vi "SCMP Rotation and Focus Check.vi"(8 "error in":errorcluster, 11 "FITS Header In":T1={"Wavelength (nm)"=530.15, "Exposure (s)"=0.05, "Tuning Delay (ms)"=1000.0, "Beam Type (-1/1)"=1.0, "Tuning Voltages"=[1.111, 2.222, 3.333, 4.444], "Observer"="observer", "Light Shapping Diffuser"=enum."In Beam", "Comment"="", "Data Type"=enum."HOLE", "Mod Cycles"=0, "SCD Calibration Optics"=enum."1 - Polarizer @0, I+Q", "SCD Emission Line Filter"=enum."1-557.6nm", "Cookbook"="", "COMP-S Calibration Wheel"=enum."Dark", "COMP-S Andover Filter Wheel"=enum."530.3nm/HWB 0.34nm (Fe XIV)", "FOV Rotation (deg)"=66.0, "Objective Lens Position (mm)"=0.0, "Occulter size"=0.0, "Time End"=timestamp(3382374145.421875 s since 1904-01-01), "Acc Exposure (s)"=0.0, "Time Stamp Array"=[], "Camera Serial Number"=[], "Camera Temp"=[], "Camera PI (mm)"=[], "Time Start"=timestamp(3382374145.421875 s since 1904-01-01), "Peripherals"={"ILX controler"=FALSE, "Zone temperatures"=FALSE, "Andor"=FALSE, "Andor 2"=FALSE, "PI Stages"=FALSE, "AISAS mechanisms"=FALSE, "AISAS Mech.lvclass"=refnum, "Zone temp ref"=variant, "FWs"=FALSE}, "FITS paths"=[], "Cameras"=enum."Andor", "load preset cbk"=FALSE, "periodic check count"=0, "COMP-S Calibration Wheel 2"=enum."Dark", "Calib"=enum."Dark", "Abso Aperture"=66.0, "Nominal Aperture"=66.0, "Pointer IP"="127.0.0.1"} {"Nominal Aperture" format="%.1f"; "Abso Aperture" format="%.1f"; "Camera PI (mm)" format="%_3g"; "Acc Exposure (s)" format="%^.3g"; "Occulter size" format="%.2f"; "Objective Lens Position (mm)" min=70.0 max=152.0 format="%.2f"; "FOV Rotation (deg)" format="%.1f"; "Exposure (s)" format="%^.3g"; "Wavelength (nm)" format="%_6g"}) -> (0 "error out":errorcluster, 1 "Comment out":string="Test", 2 "Observer out":string="Observer", 3 "FITS Header Out":T1={"Wavelength (nm)"=530.15, "Exposure (s)"=0.05, "Tuning Delay (ms)"=1000.0, "Beam Type (-1/1)"=1.0, "Tuning Voltages"=[1.111, 2.222, 3.333, 4.444], "Observer"="observer", "Light Shapping Diffuser"=enum."In Beam", "Comment"="", "Data Type"=enum."HOLE", "Mod Cycles"=0, "SCD Calibration Optics"=enum."1 - Polarizer @0, I+Q", "SCD Emission Line Filter"=enum."1-557.6nm", "Cookbook"="", "COMP-S Calibration Wheel"=enum."Dark", "COMP-S Andover Filter Wheel"=enum."530.3nm/HWB 0.34nm (Fe XIV)", "FOV Rotation (deg)"=66.0, "Objective Lens Position (mm)"=0.0, "Occulter size"=0.0, "Time End"=timestamp(3382374145.421875 s since 1904-01-01), "Acc Exposure (s)"=0.0, "Time Stamp Array"=[], "Camera Serial Number"=[], "Camera Temp"=[], "Camera PI (mm)"=[], "Time Start"=timestamp(3382374145.421875 s since 1904-01-01), "Peripherals"={"ILX controler"=FALSE, "Zone temperatures"=FALSE, "Andor"=FALSE, "Andor 2"=FALSE, "PI Stages"=FALSE, "AISAS mechanisms"=FALSE, "AISAS Mech.lvclass"=refnum, "Zone temp ref"=variant, "FWs"=FALSE}, "FITS paths"=[], "Cameras"=enum."Andor", "load preset cbk"=FALSE, "periodic check count"=0, "COMP-S Calibration Wheel 2"=enum."Dark", "Calib"=enum."Dark", "Abso Aperture"=66.0, "Nominal Aperture"=66.0, "Pointer IP"="127.0.0.1"} {"Nominal Aperture" format="%.1f"; "Abso Aperture" format="%.1f"; "Camera PI (mm)" format="%_3g"; "Acc Exposure (s)" format="%^.3g"; "Occulter size" format="%.2f"; "Objective Lens Position (mm)" min=70.0 max=152.0 format="%.2f"; "FOV Rotation (deg)" format="%.1f"; "Exposure (s)" format="%^.3g"; "Wavelength (nm)" format="%_6g"}, 5 "Pointer IP":string)   [LabVIEW 2014]
uses:
  Controls/Diffuser.ctl
  Controls/SCMP observers.ctl
  Controls/SCD - FITS Cluster.ctl
  Mech/AISAS Mech.lvclass
  Controls/FITS Data type.ctl
  Controls/SCD - Calibration Optics Filter Wheel.ctl
  Controls/SCD - EDT - Emission Line Filter Wheel.ctl
  Controls/CoMP-S Controls/Polarization Optics Filter Wheel.ctl
  Controls/CoMP-S Controls/Emission Line Filter Wheel.ctl
  Controls/focus.ctl
  Controls/peripherals.ctl
  Controls/Cameras select.ctl
  <vilib>/Utility/xml.llb/Read From XML File(array).vi
panel:
  in  "Nominal Aperture":dbl=196.0 caption="Nominal aperture diameter [mm]" min=0.0 max=360.0 format="%.1f"
  in  "Abs Aperture":dbl=39.7 caption="Absolute calibration aperture diameter [mm]" min=0.0 max=360.0 format="%.1f"
  in  "Focus":dbl=103.0 min=70.0 max=152.0 format="%.2f"
  in  "Occulter size":dbl=103.0 format="%.2f"
  out "Generated XML":string
  in  "Observer":string="Observer"
  in  "Comment":string="Test"
  in  "Observer Enum":T11 items=["INY", "RYBAK", "SCHWARTZ", "HUTAR", "TREMBAC"]
  in  "Diffuser":T2=enum."In Beam"
  out "OBS_PROG OUT":string
  in  "Observer Program":u16(ring) items=["TEST", "OBS_PROG 001: SPEKTROPOLARIMETRIA POKOJNEJ PROTUBERANCIE A JEJ KAVITY - 854,656,637,530 (P.Schwartz)", "OBS_PROG 002: SPEKTROPOLARIMETRIA POKOJNEJ PROTUBERANCIE - 656 (Y.Su)", "OBS_PROG 003: SPEKTROPOLARIMETRIA PROTUBERANCII A KORONY - 656,587,530 (P.Schwartz)", "OBS_PROG 004: SPEKTROPOLARIMETRIA FILAMENTOV NA DISKU - 854,656,587 (P.Schwartz)", "OBS_PROG 005: SPEKTROPOLARIMETRIA PROTUBERANCII -s 854,656,587,530 (P.Schwartz)", "OBS_PROG 006: SPEKTROPOLARIMETRIA PROTUBERANCII A KORONY - 854,656,587,530 (P.Schwartz)", "CAL_PROG 001: CORONAGRAPH FOCUS DETERMINATION FOR ALL LINES", "TEST_PROG 001: DATA ACQUISITION BY CAMERAS"]
  out "Observer txt":string
  in  "Rotation Angle":dbl min=0.0 max=360.0 format="%.1f"
  in  "stop":bool
  # "Please check initial values !!!"
  # "motorized 39.7 mm, manual 40.0 mm"
  # "If values are right, then press OK"
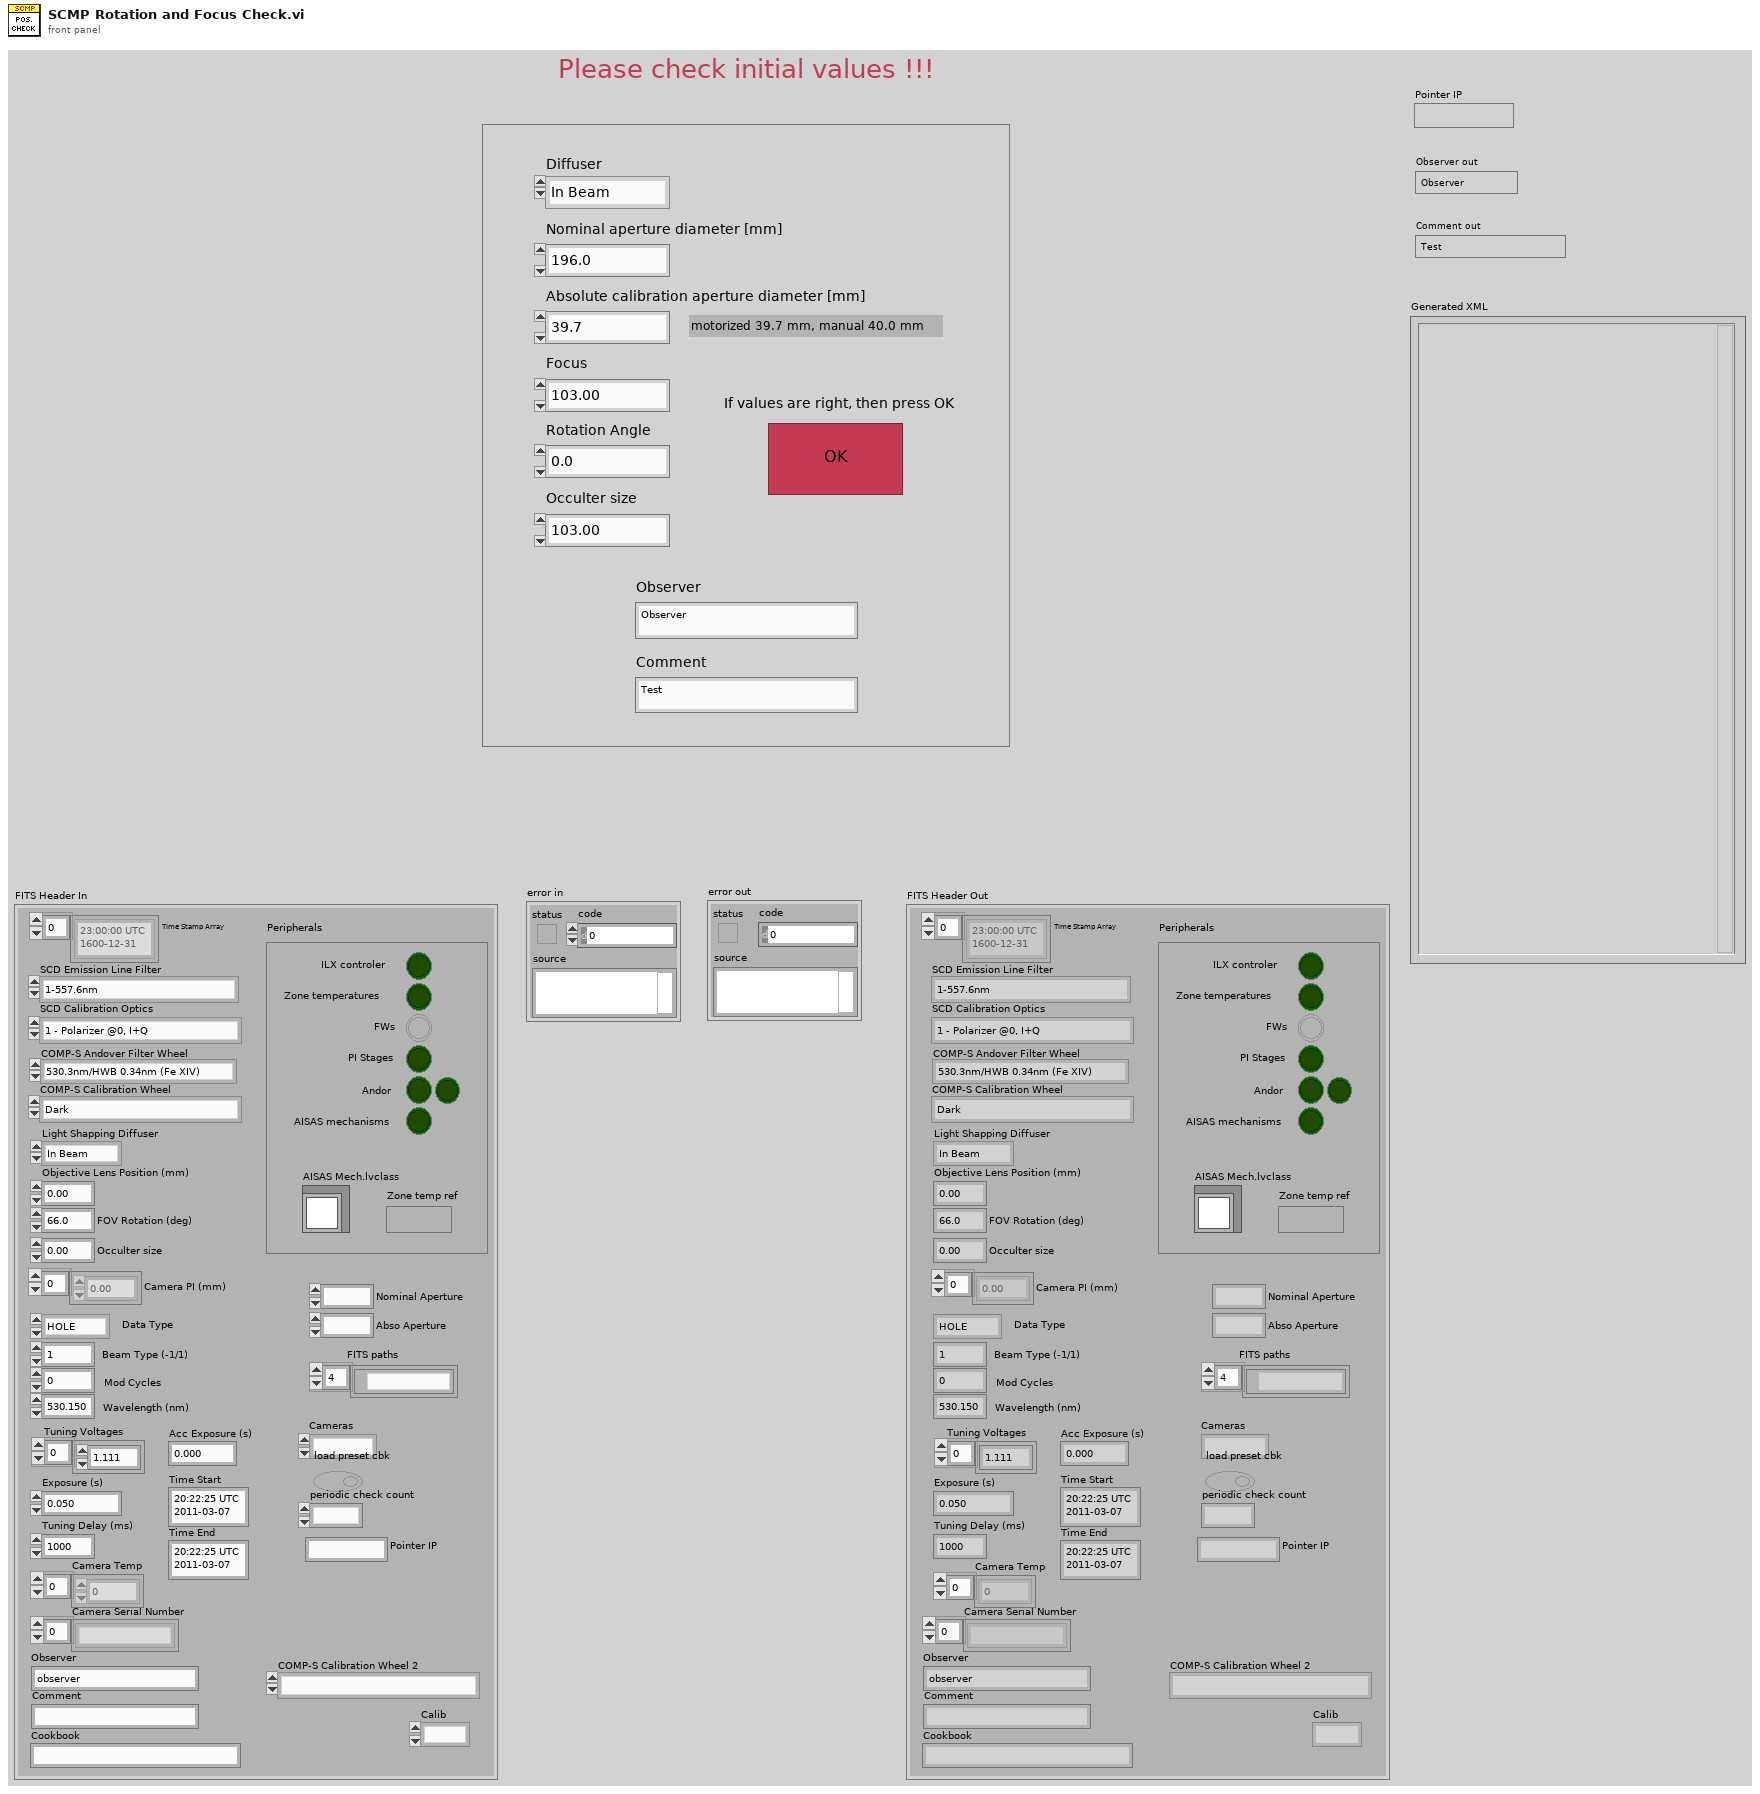
[diagram p1: front panel]
types:
  T1 = typedef "SCD - FITS Cluster.ctl" = cluster{"Wavelength (nm)":dbl, "Exposure (s)":dbl, "Tuning Delay (ms)":dbl, "Beam Type (-1/1)":dbl, "Tuning Voltages":dbl[], "Observer":string, "Light Shapping Diffuser":T2, "Comment":string, "Data Type":T3, "Mod Cycles":u16, "SCD Calibration Optics":T4, "SCD Emission Line Filter":T5, "Cookbook":string, "COMP-S Calibration Wheel":T6, "COMP-S Andover Filter Wheel":T7, "FOV Rotation (deg)":dbl, "Objective Lens Position (mm)":T8, "Occulter size":dbl, "Time End":timestamp, "Acc Exposure (s)":dbl, "Time Stamp Array":timestamp[], "Camera Serial Number":string[], "Camera Temp":dbl[], "Camera PI (mm)":dbl[], "Time Start":timestamp, "Peripherals":T9, "FITS paths":path[], "Cameras":T10, "load preset cbk":bool, "periodic check count":i32, "COMP-S Calibration Wheel 2":T6, "Calib":enum16{"Dark", "Flat"}, "Abso Aperture":dbl, "Nominal Aperture":dbl, "Pointer IP":string}
  T2 = typedef "Diffuser.ctl" = enum16{"Out of Beam", "In Beam"}
  T3 = typedef "FITS Data type.ctl" = enum16{"LIVE", "DARK", "FLAT", "CALI", "OBSE", "ABSO", "AURE", "TARG", "OBJE", "HOLE", "OREX", "THRO", "CHIP"}
  T4 = typedef "SCD - Calibration Optics Filter Wheel.ctl" = enum16{"1 - Polarizer @0, I+Q", "2 - Polarizer @90, I-Q", "3 - Polarizer @45, I+U", "4 - Polarizer @135, I-U", "5 - Polarizer @0, Retarder @45, I+V", "6 - Polarizer @0, Retarder @135, I-V", "7 - Dark", "8 - Clear", "9 - N/A"}
  T5 = typedef "SCD - EDT - Emission Line Filter Wheel.ctl" = enum16{"1-557.6nm", "2-587.6nm", "3-589.6nm", "4-630.2nm", "5-656.4nm", "6-849.8nm", "7-854.2nm", "8-866.2nm", "9-1083.0nm"}
  T6 = typedef "Polarization Optics Filter Wheel.ctl" = enum16{"Dark", "Clear", "Exchange Lens", "Polarizer @0, I+Q", "Polarizer @90, I-Q", "Polarizer @45, I+U", "Polarizer @135, I-U", "Polarizer @0, Retarder @45, I+V", "Polarizer @0, Retarder @135, I-V"}
  T7 = typedef "Emission Line Filter Wheel.ctl" = enum16{"530.3nm/HWB 0.34nm (Fe XIV)", "587.6nm/HBW 0.44nm (He I D3)", "637.5nm/HBW 0.53nm (Fe X)", "656.3nm/HBW 0.57nm (H-Alpha)", "789.2nm/HBW 0.85nm (Fe XI)", "854.2nm/HBW 1.01nm (Ca I)", "1074.7nm/HBW 2.34nm (Fe XIII)", "1079.8nm/HBW 1.64nm (Fe XIII)", "1083.0nm/HBW 1.66nm (He I)"}
  T8 = typedef "focus.ctl" = dbl
  T9 = typedef "peripherals.ctl" = cluster{"ILX controler":bool, "Zone temperatures":bool, "Andor":bool, "Andor 2":bool, "PI Stages":bool, "AISAS mechanisms":bool, "AISAS Mech.lvclass":refnum<class "AISAS Mech.lvclass">, "Zone temp ref":variant, "FWs":bool}
  T10 = typedef "Cameras select.ctl" = enum16{"Andor", "GDR"}
  T11 = typedef "SCMP observers.ctl" = u16
  T12 = enum8{"Enabled", "Disabled", "Disabled and Grayed Out"}
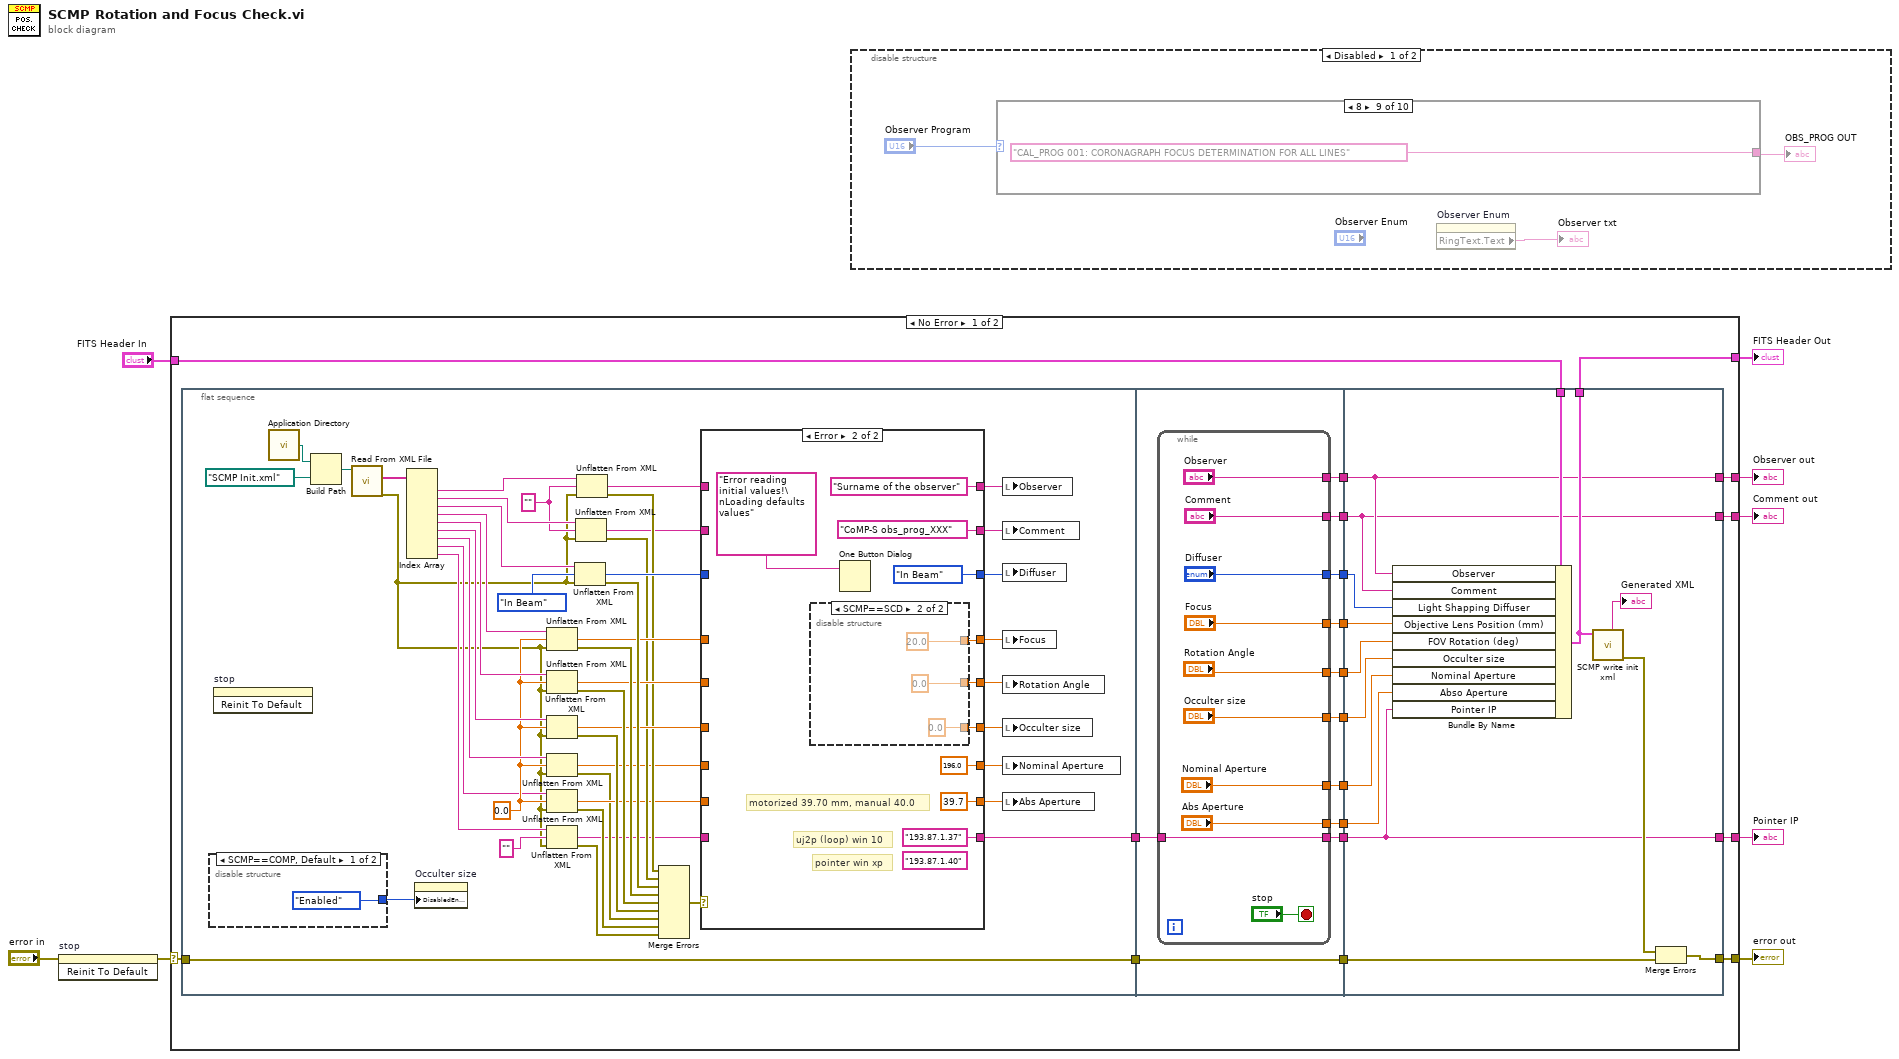
[diagram p0: block diagram]
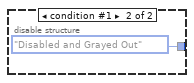
[diagram p2: hidden frame]
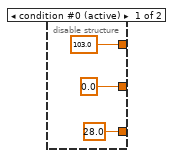
[diagram p4: hidden frame]
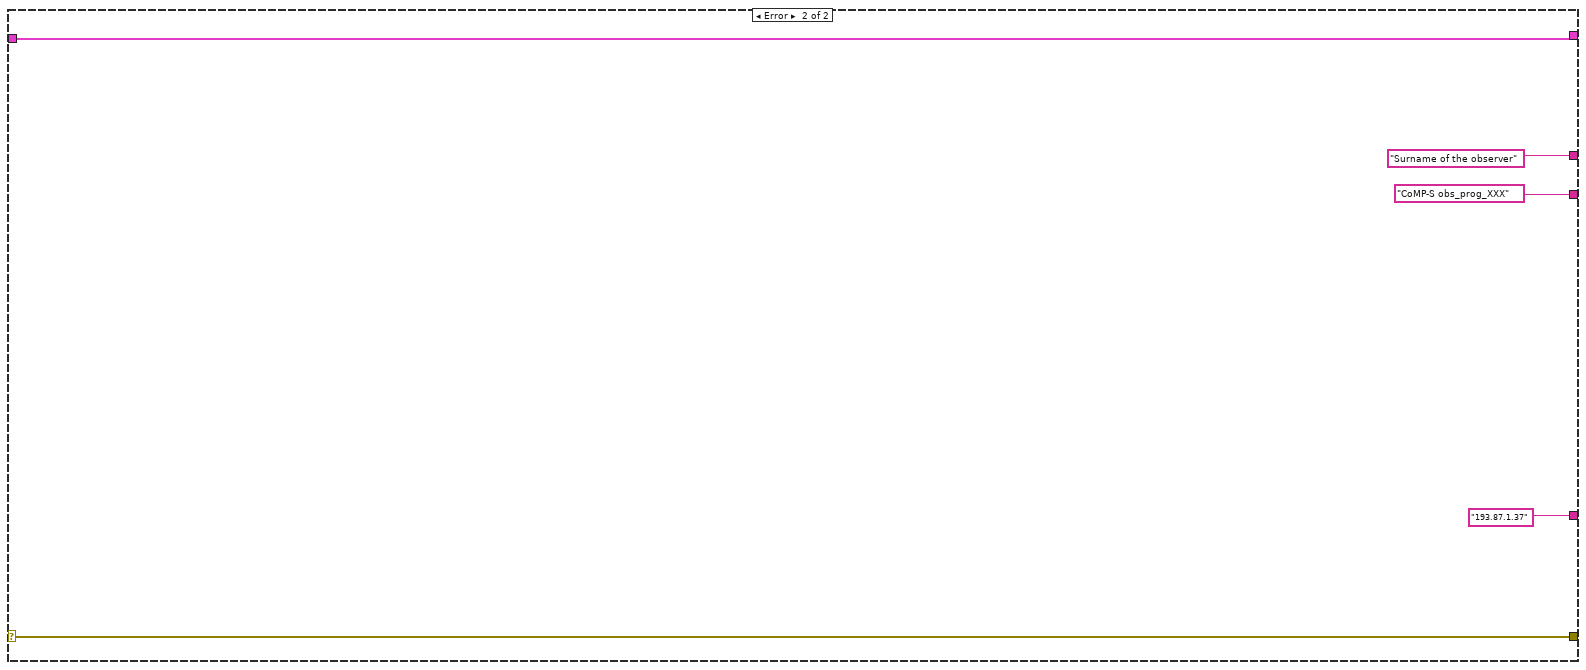
[diagram p5: hidden frame]
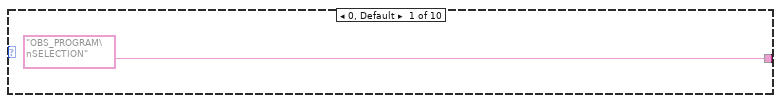
[diagram p6: hidden frame]
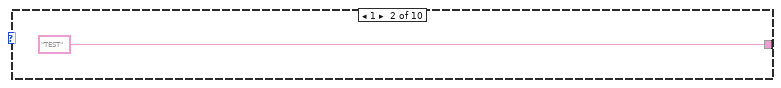
[diagram p7: hidden frame]
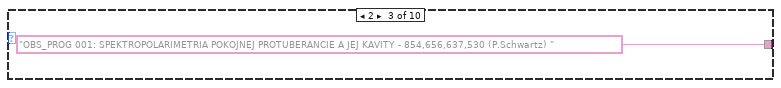
[diagram p8: hidden frame]
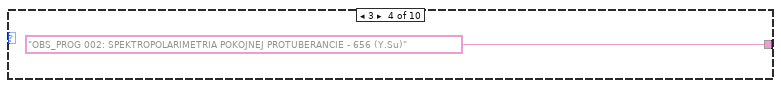
[diagram p9: hidden frame]
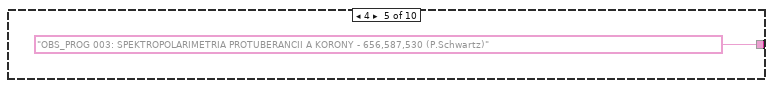
[diagram p10: hidden frame]
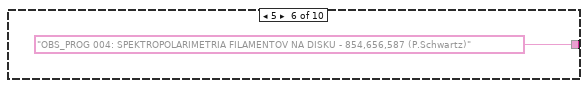
[diagram p11: hidden frame]
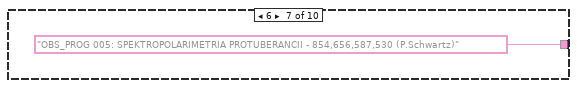
[diagram p12: hidden frame]
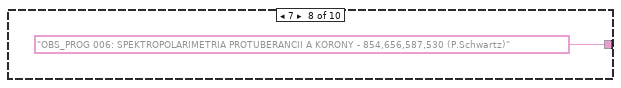
[diagram p13: hidden frame]
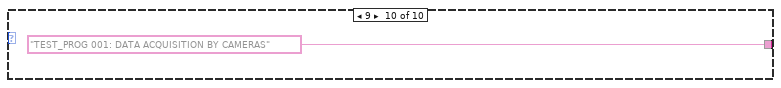
[diagram p14: hidden frame]
diagram:
  n1 = invoke on="stop" class="Bool" method="Reinit To Default"(error in="error in") -> (error out=w4:errorcluster)  [unwired: 2 in, 2 out]
  n2 = case shown="No Error" w4 {
    selector: w4 -> [w18 w143]
    tunnel: [w19 w143] -> w8
    tunnel: "FITS Header In" -> [w17 w142]
    tunnel: [w16 w142] -> w6
    tunnel: [w15 "Surname of the observer" ("element")] -> w3
    tunnel: [w14 "CoMP-S obs_prog_XXX" ("element")] -> w2
    tunnel: [w9 "193.87.1.37" ("element")] -> w1
    frame No Error {
      n3 = flat-sequence {
        tunnel: [w62] -> w27
        tunnel: w18 -> [w62]
        tunnel: [w29] -> w10
        tunnel: [w113] -> w26
        tunnel: [w112] -> w25
        tunnel: [w111] -> w24
        tunnel: [w110] -> w23
        tunnel: [w109] -> w22
        tunnel: [w108] -> w21
        tunnel: [w107] -> w20
        tunnel: w27 -> [w107]
        tunnel: [w106] -> w13
        tunnel: [w105] -> w12
        tunnel: [w104] -> w11
        tunnel: w10 -> [w103]
        tunnel: w26 -> [w133]
        tunnel: w25 -> [w132]
        tunnel: w24 -> [w127]
        tunnel: w23 -> [w129]
        tunnel: w22 -> [w128]
        tunnel: w21 -> [w131]
        tunnel: [w136] -> w19
        tunnel: w20 -> [w137]
        tunnel: w17 -> [w134]
        tunnel: [w130] -> w16
        tunnel: [w129] -> w15
        tunnel: [w128] -> w14
        tunnel: w13 -> [w126]
        tunnel: w12 -> [w125]
        tunnel: w11 -> [w124]
        tunnel: [w124] -> w9
        frame #0 {
          w48 = "" ("element")
          w39 = 0.0 ("Mean")
          n4 = disable-structure shown="SCMP==COMP, Default" {
            disable-tunnel: [T12."Enabled" ("Disabled") T12."Disabled and Grayed Out" ("Disabled")] -> w57
            frame condition #0 (active) {
            }
            frame condition #1 {
            }
          }
          n5 = invoke on="stop" class="Bool" method="Reinit To Default"() -> ()  [unwired: 3 in, 3 out]
          n6 = call <vilib>:"Application Directory.vi"() -> ("Application Directory"=w74:path)
          n7 = Build Path(base path=w74, name or relative path=path "SCMP Init.xml" ("default name")) -> (appended path=w58:path)
          n8 = call-poly <vilib>:"Read From XML File.vi"("XML File Path"=w58) -> ("error out"=w30:errorcluster, "XML Elements"=w68:string[])  [unwired: 8 in, 1 out]
          n9 = Index Array(array=w68) -> (element #1=w51:string, element #2=w52:string, element #3=w53:string, element #4=w54:string, element #5=w55:string, element #6=w56:string, element #7=w43:string, element #8=w38:string, element #9=w31:string)  [unwired: 9 in]
          n10 = property on="Occulter size" class="DigNum (strict)"("DisabledEnum"=w57) -> ()  [unwired: 2 in, 2 out]
          n11 = Unflatten From XML(xml string=w54, type=w39, error in (no error)=w30) -> (value=w66:dbl, error out=w70:errorcluster)
          n12 = Unflatten From XML(xml string=w55, type=w39, error in (no error)=w30) -> (value=w65:dbl, error out=w69:errorcluster)
          n13 = Unflatten From XML(xml string=w56, type=w39, error in (no error)=w30) -> (value=w63:dbl, error out=w42:errorcluster)
          n14 = Unflatten From XML(xml string=w43, type=w39, error in (no error)=w30) -> (value=w41:dbl, error out=w35:errorcluster)
          n15 = Unflatten From XML(xml string=w38, type=w39, error in (no error)=w30) -> (value=w36:dbl, error out=w34:errorcluster)
          n16 = Unflatten From XML(xml string=w31, type="" ("element"), error in (no error)=w30) -> (value=w28:string, error out=w33:errorcluster)
          n17 = Unflatten From XML(xml string=w53, type=Diffuser."In Beam" ("Diffuser"), error in (no error)=w30) -> (value=w67:T2, error out=w71:errorcluster)
          n18 = Unflatten From XML(xml string=w52, type=w48, error in (no error)=w30) -> (value=w44:string, error out=w50:errorcluster)
          n19 = Unflatten From XML(xml string=w51, type=w48, error in (no error)=w30) -> (value=w47:string, error out=w49:errorcluster)
          n20 = Merge Errors(w49, w50, w71, w70, w69, w42, w35, w34, w33) -> (w59:errorcluster)
          n21 = case shown="Error" w59 {
            tunnel: [w84 w93] -> w73
            tunnel: [w86 Diffuser."In Beam" ("Diffuser")] -> w60
            tunnel: [w85 w94] -> w72
            tunnel: w67 -> [w86 _]
            tunnel: w66 -> [w85 _]
            tunnel: w65 -> [w84 _]
            tunnel: [w83 w92] -> w64
            tunnel: w63 -> [w83 _]
            tunnel: w47 -> [w82 _]
            tunnel: [w82 "Surname of the observer" ("element")] -> w46
            tunnel: [w81 "CoMP-S obs_prog_XXX" ("element")] -> w45
            tunnel: w44 -> [w81 _]
            tunnel: w41 -> [w80 _]
            tunnel: [w80 196.0 ("Mean")] -> w40
            tunnel: [w79 39.7 ("Mean")] -> w37
            tunnel: w36 -> [w79 _]
            tunnel: [w78 "193.87.1.37" ("element")] -> w29
            tunnel: w28 -> [w78 _]
            frame No Error {
            }
            frame Error {
              (unwired) "193.87.1.40" ("element")
              # "motorized 39.70 mm, manual 40.0"
              # "pointer win xp"
              # "uj2p (loop) win 10"
              n22 = disable-structure shown="SCMP==SCD" {
                disable-tunnel: [103.0 ("Mean") 20.0 ("Mean")] -> w94
                disable-tunnel: [0.0 0.0] -> w93
                disable-tunnel: [28.0 ("Mean") 0.0 ("Mean")] -> w92
                frame condition #0 (active) {
                }
                frame condition #1 {
                }
              }
              n23 = One Button Dialog(message="Error reading initial values!\nLoading defaults values" ("error source (\" \")")) -> ()  [unwired: 1 in, 1 out]
            }
          }
          n24 = local write "Observer"(w46) -> ()
          n25 = local write "Comment"(w45) -> ()
          n26 = local write "Diffuser"(w60) -> ()
          n27 = local write "Focus"(w72) -> ()
          n28 = local write "Rotation Angle"(w73) -> ()
          n29 = local write "Occulter size"(w64) -> ()
          n30 = local write "Nominal Aperture"(w40) -> ()
          n31 = local write "Abs Aperture"(w37) -> ()
        }
        frame #1 {
          n32 = while {
            tunnel: ["Focus"] -> w113
            tunnel: ["Rotation Angle"] -> w112
            tunnel: ["Diffuser"] -> w111
            tunnel: ["Observer"] -> w110
            tunnel: ["Comment"] -> w109
            tunnel: ["Occulter size"] -> w108
            tunnel: ["Nominal Aperture"] -> w106
            tunnel: ["Abs Aperture"] -> w105
            tunnel: [w114] -> w104
            tunnel: w103 -> [w114]
            stop <- "stop" stop-if-true
          }
        }
        frame #2 {
          n33 = Bundle By Name(cluster=w134, "Observer"=w129, "Comment"=w128, "Light Shapping Diffuser"=w127, "Objective Lens Position (mm)"=w133, "FOV Rotation (deg)"=w132, "Occulter size"=w131, "Nominal Aperture"=w126, "Abso Aperture"=w125, "Pointer IP"=w124) -> (w130:T1)
          n34 = call "SCMP write init xml.vi"("FITS Header In"=w130) -> ("error out"=w135:errorcluster, "XML String"=→"Generated XML":string)  [unwired: 9 in]
          n35 = Merge Errors(w135, w137) -> (w136:errorcluster)
        }
      }
    }
    frame Error {
    }
  }
  "error out" <- w8
  "FITS Header Out" <- w6
  "Observer out" <- w3
  "Comment out" <- w2
  "Pointer IP" <- w1
  n36 = disable-structure shown="Disabled" {
    frame Disabled {
      n37 = case shown="8" "Observer Program" {
        tunnel: ["OBS_PROGRAM\nSELECTION" "TEST" "OBS_PROG 001: SPEKTROPOLARIMETRIA POKOJNEJ PROTUBERANCIE A JEJ KAVITY - 854,656,637,530 (P.Schwartz) " "OBS_PROG 002: SPEKTROPOLARIMETRIA POKOJNEJ PROTUBERANCIE - 656 (Y.Su)" "OBS_PROG 003: SPEKTROPOLARIMETRIA PROTUBERANCII A KORONY - 656,587,530 (P.Schwartz)" "OBS_PROG 004: SPEKTROPOLARIMETRIA FILAMENTOV NA DISKU - 854,656,587 (P.Schwartz)" "OBS_PROG 005: SPEKTROPOLARIMETRIA PROTUBERANCII - 854,656,587,530 (P.Schwartz)" "OBS_PROG 006: SPEKTROPOLARIMETRIA PROTUBERANCII A KORONY - 854,656,587,530 (P.Schwartz)" "CAL_PROG 001: CORONAGRAPH FOCUS DETERMINATION FOR ALL LINES" "TEST_PROG 001: DATA ACQUISITION BY CAMERAS"] -> w144
        frame 0, Default {
        }
        frame 1 {
        }
        frame 2 {
        }
        frame 3 {
        }
        frame 4 {
        }
        frame 5 {
        }
        frame 6 {
        }
        frame 7 {
        }
        frame 8 {
        }
        frame 9 {
        }
      }
      "OBS_PROG OUT" <- w144
      n38 = property on="Observer Enum" class="Ring (strict)"() -> ("RingText.Text"=→"Observer txt":string)  [unwired: 2 in, 2 out]
    }
    frame Enabled {
    }
  }
